vi "Read QObject Class Ref.vi"(8 "error in (no error)":errorcluster, 11 "QObject Writer in":refnum<class "QObject Writer.lvclass">) -> (0 "error out":errorcluster, 2 "QObject Class Ref":refnum<vi>, 3 "QObject Writer out":refnum<class "QObject Writer.lvclass">)   [LabVIEW 2013, in "QObject Writer.lvclass"]
uses:
  QObject Writer.lvclass
  QObject Writer.lvclass/QObject Writer.ctl
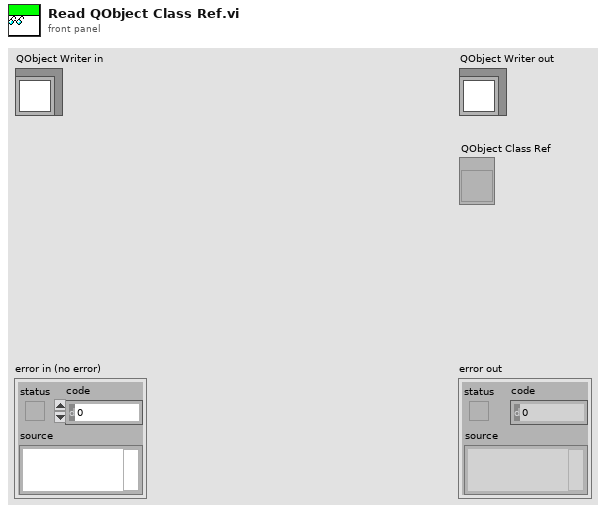
[diagram p1: front panel]
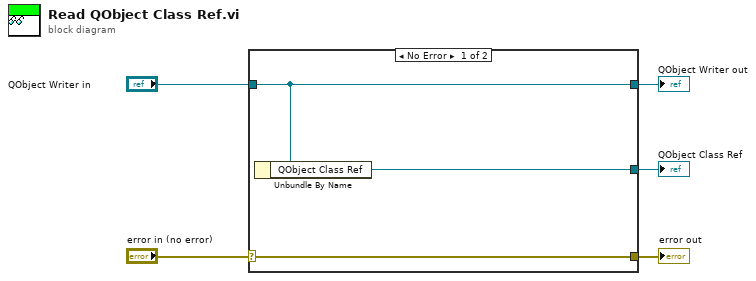
[diagram p0: block diagram]
diagram:
  n1 = case shown="No Error" "error in (no error)" {
    selector: "error in (no error)" -> [w8 w9]
    tunnel: [w8 w9] -> w4
    tunnel: [w7 w10] -> w2
    tunnel: "QObject Writer in" -> [w7 w10]
    tunnel: [w6 _] -> w1
    frame No Error {
      n2 = Unbundle By Name(w7) -> ("QObject Class Ref"=w6:refnum<vi>)
    }
    frame Error {
    }
  }
  "error out" <- w4
  "QObject Writer out" <- w2
  "QObject Class Ref" <- w1
